vi "WIP_Rearrange.vi"(11 "WIP in":i64[](array[numeric])) -> (3 "WIP out":i64[](array[numeric]))   [LabVIEW 2020]
uses:
  MS SQL/MS_Global.vi
  <userlib>/_OpenG.lib/array/array.llb/Search 1D Array (Boolean)__ogtk.vi
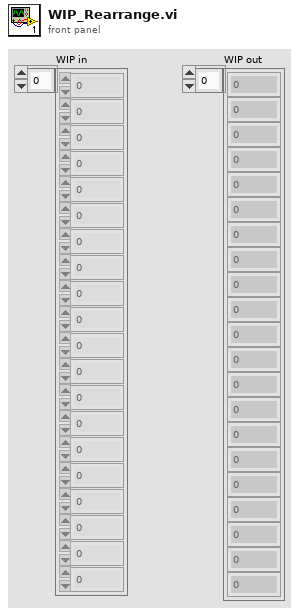
[diagram p1: front panel]
types:
  T1 = typedef "WIP_ref.ctl" = cluster{"WIP 1":refnum<vi>, "WIP 2":refnum<vi>, "WIP 3":refnum<vi>}
  T2 = cluster{"WIP Ref[0]":refnum<vi>, "WIP Ref[1]":refnum<vi>, "WIP Ref[2]":refnum<vi>}
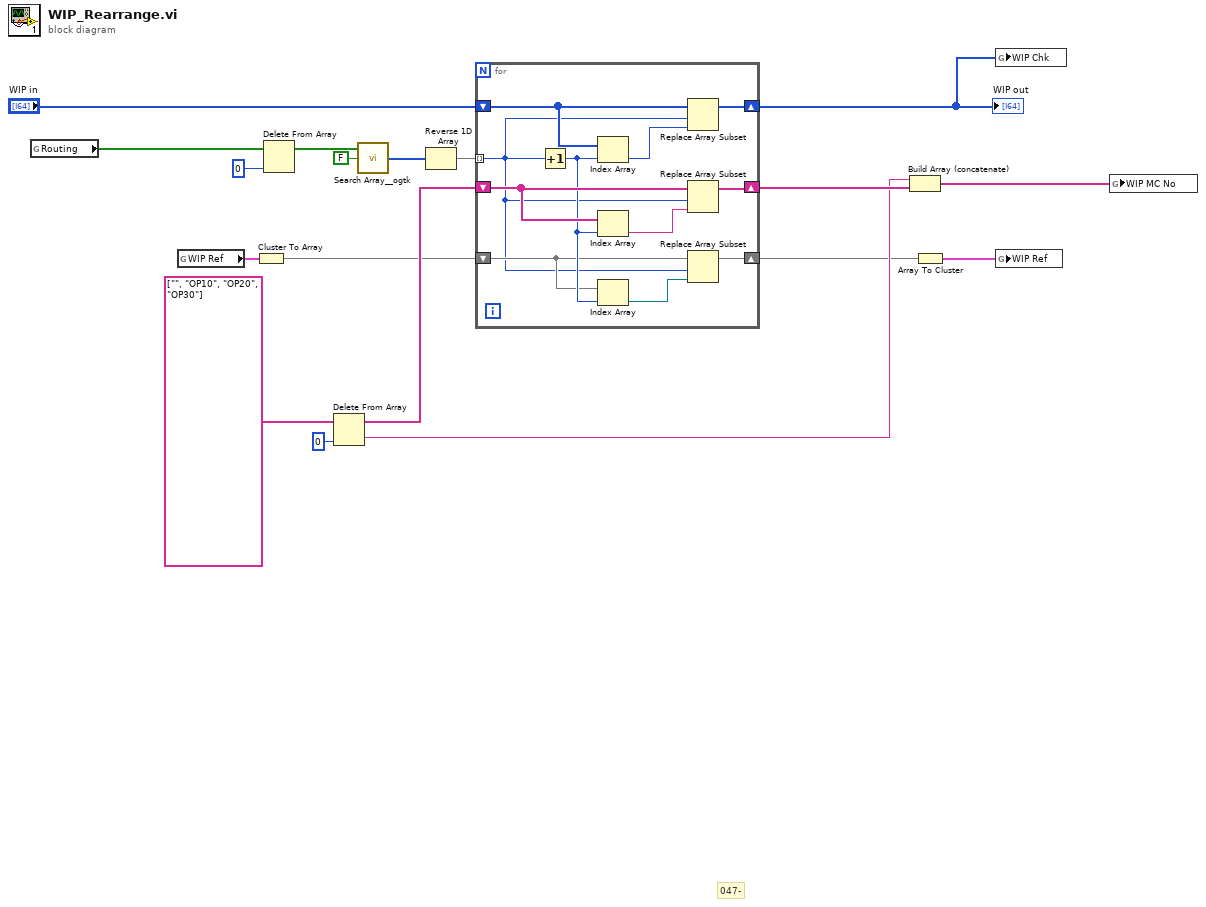
[diagram p0: block diagram]
diagram:
  # "047-"
  n1 = global read "MS_Global.vi" "Routing"() -> (w12:bool[])
  n2 = global read "MS_Global.vi" "WIP Ref"() -> (w5:T1)
  n3 = Cluster To Array(cluster=w5) -> (array=w4:refnum<vi>[])
  n4 = Delete From Array(array=w12, index=0) -> (array with subset deleted=w11:bool[])  [unwired: 1 in, 1 out]
  n5 = Delete From Array(array=string[] ["", "OP10", "OP20", "OP30"] ("TS_CODE_TAG"), index=0) -> (deleted portion=w6:string, array with subset deleted=w8:string[])  [unwired: 1 in]
  n6 = call-poly <userlib>:"Search Array__ogtk.vi"("Array"=w11, "Element Data"=FALSE) -> ("Indices of Elements"=w15:i32[])  [unwired: 7 in]
  n7 = Reverse 1D Array(array=w15) -> (reversed array=w14:i32[])
  n8 = for {
    tunnel: w14 -> [w19] mode=indexing
    shift-right: [w28] -> w1
    shift-left: "WIP in" -> [w29]
    shift-right: [w24] -> w9
    shift-left: w8 -> [w26]
    shift-right: [w21] -> w3
    shift-left: w4 -> [w22]
    n9 = Increment(x=w19) -> (x+1=w23:i32)
    n10 = Index Array(array=w29, index=w23) -> (element=w27:i64)
    n11 = Index Array(array=w26, index=w23) -> (element=w25:string)
    n12 = Index Array(array=w22, index=w23) -> (element=w20:refnum<vi>)
    n13 = Replace Array Subset(array=w29, new element=w27, index=w19) -> (w28:i64[])
    n14 = Replace Array Subset(array=w26, new element=w25, index=w19) -> (w24:string[])
    n15 = Replace Array Subset(array=w22, new element=w20, index=w19) -> (w21:refnum<vi>[])
  }
  "WIP out" <- w1
  n16 = Build Array (concatenate)(w6, w9) -> (w7:string[])
  n17 = Array To Cluster(array=w3) -> (cluster=w2:T2)
  n18 = global write "MS_Global.vi" "WIP Chk"(w1) -> ()
  n19 = global write "MS_Global.vi" "WIP Ref"(w2) -> ()
  n20 = global write "MS_Global.vi" "WIP MC No"(w7) -> ()
